vi "Close.vi"(8 "error in (no error)":errorcluster, 11 "REST_Client in":refnum<class "REST_Client.lvclass">) -> (0 "error out":errorcluster)   [LabVIEW 2020, in "REST_Client.lvclass"]
uses:
  REST_Client.lvclass
  <vilib>/httpClient/LabVIEWHTTPClient.lvlib
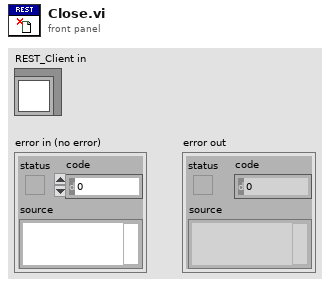
[diagram p1: front panel]
types:
  T1 = typedef "LabVIEWHTTPClient.lvlib/ClientHandle.ctl" = refnum<k1>
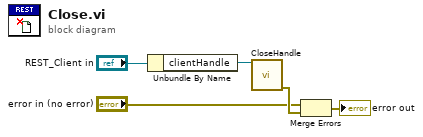
[diagram p0: block diagram]
diagram:
  n1 = Unbundle By Name("REST_Client in") -> ("clientHandle"=w4:T1)
  n2 = call <vilib>:"CloseHandle.vi"("client handle"=w4) -> ("error out"=w3:errorcluster)  [unwired: 14 in]
  n3 = Merge Errors("error in (no error)", w3) -> (→"error out":errorcluster)
